vi "Create All Message Queues.vi"(8 "error in (no error)":errorcluster, 11 "Process Name":string) -> (0 "error out":errorcluster, 3 "Message Queues":T1)   [LabVIEW 2018, in "Feed Module.lvlib"]
uses:
  Feed Module.lvlib
  Controls/Feed Message Queues.ctl
  support/Message Queue/Message Cluster.ctl
  Config Module/Controls/OP Window Display.ctl
  Controls/Feed Module Display.ctl
  Measure Instrument/PID Input Enum.ctl
  Measure Instrument/PID 2 Output Enum.ctl
  support/Message Queue/Enqueue Message (Single).vi
  support/Message Queue/Message Queue.lvlib
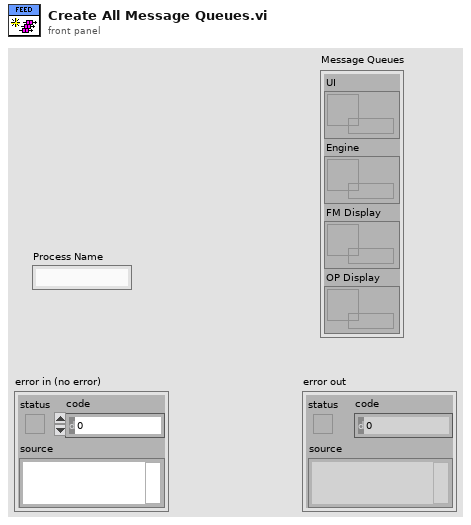
[diagram p1: front panel]
types:
  T1 = typedef "Feed Module.lvlib/Feed Message Queues.ctl" = cluster{"UI":refnum<queue>, "Engine":refnum<queue>, "FM Display":refnum<queue>, "OP Display":refnum<queue>}
  T2 = typedef "Feed Module.lvlib/Feed Module Display.ctl" = cluster{"Flow":dbl, "Density":dbl, "FL Temp":dbl, "Scale Value":dbl, "Pump On?":enum16{"Off", "On", "Not Initialized"}, "Cycle Period":dbl, "Input Device":T3, "Output":T4, "Pump's Pressure":dbl, "Pump's Flow ":dbl}
  T3 = typedef "PID Input Enum.ctl" = enum16{"Default", "Bronkhorst M13", "Bronkhorst M14", "Scale Rate of Change"}
  T4 = typedef "PID 2 Output Enum.ctl" = enum16{"Default", "Ismatec ISM 4308", "Ismatec ISM 831C", "Masterflex 7550-30", "VICI", "Tacmina QI", "KNF SIMDOS", "ASIA Type C", "FLOM UI-22-11", "SSI PR/LD", "SSI P40", "Masterflex 75211-70"}
  T5 = typedef "Feed Module.lvlib/OP Window Display.ctl" = cluster{"Flow":dbl, "Manual":dbl, "Pump Status":u16, "Smoothed Array":dbl[]}
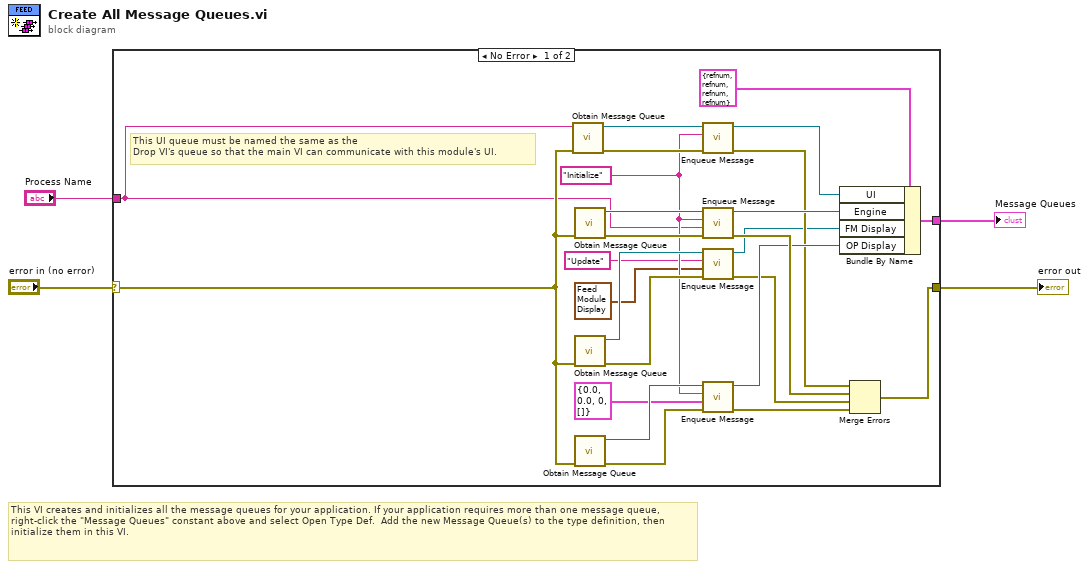
[diagram p0: block diagram]
diagram:
  # "This VI creates and initializes all the message queues for your application. If your application requires more than one message queue, right-click the \"Message Queues\" constant above and select Open Type Def.  Add the new Message Queue(s) to the type definition, then initialize them in this VI."
  n1 = case shown="No Error" "error in (no error)" {
    selector: "error in (no error)" -> [w15 w30]
    tunnel: [w26 w30] -> w4
    tunnel: [w29 _] -> w3
    tunnel: "Process Name" -> [w5 _]
    frame No Error {
      w12 = "Initialize" ("Message")
      # "This UI queue must be named the same as the \nDrop VI's queue so that the main VI can communicate with this module's UI."
      n2 = call "Obtain Message Queue.vi"("error in (no error)"=w15, "name (unnamed)"=w5) -> ("error out"=w28:errorcluster, "Message Queue"=w27:refnum<queue>)  [unwired: 8 in]
      n3 = call "Obtain Message Queue.vi"("error in (no error)"=w15) -> ("error out"=w24:errorcluster, "Message Queue"=w25:refnum<queue>)  [unwired: 9 in]
      n4 = call "Obtain Message Queue.vi"("error in (no error)"=w15) -> ("error out"=w21:errorcluster, "Message Queue"=w20:refnum<queue>)  [unwired: 9 in]
      n5 = call "Obtain Message Queue.vi"("error in (no error)"=w15) -> ("error out"=w19:errorcluster, "Message Queue"=w18:refnum<queue>)  [unwired: 9 in]
      n6 = call-poly "Enqueue Message.vi"("error in (no error)"=w28, "Message"=w12, "Message Queue"=w27) -> ("error out"=w10:errorcluster, "dup Message Queue"=w11:refnum<queue>)  [unwired: 7 in]
      n7 = call-poly "Enqueue Message.vi"("error in (no error)"=w24, "Message Data"=w5, "Message"=w12, "Message Queue"=w25) -> ("error out"=w22:errorcluster, "dup Message Queue"=w23:refnum<queue>)  [unwired: 6 in]
      n8 = call-poly "Enqueue Message.vi"("error in (no error)"=w21, "Message Data"=T2 {"Flow"=0.0, "Density"=0.0, "FL Temp"=0.0, "Scale Value"=0.0, "Pump On?"=enum."Not Initialized", "Cycle Period"=500.0, "Input Device"=enum."Default", "Output"=enum."Default", "Pump's Pressure"=0.0, "Pump's Flow "=0.0}, "Message"="Update", "Message Queue"=w20) -> ("error out"=w6:errorcluster, "dup Message Queue"=w7:refnum<queue>)  [unwired: 6 in]
      n9 = call-poly "Enqueue Message.vi"("error in (no error)"=w19, "Message Data"=T5 {"Flow"=0.0, "Manual"=0.0, "Pump Status"=0, "Smoothed Array"=[]}, "Message"=w12, "Message Queue"=w18) -> ("error out"=w13:errorcluster, "dup Message Queue"=w16:refnum<queue>)  [unwired: 6 in]
      n10 = Bundle By Name(cluster=T1 {"UI"=refnum, "Engine"=refnum, "FM Display"=refnum, "OP Display"=refnum} ("Message Queues"), "UI"=w11, "Engine"=w23, "FM Display"=w7, "OP Display"=w16) -> (w29:T1)
      n11 = Merge Errors(w10, w22, w6, w13) -> (w26:errorcluster)
    }
    frame Error {
    }
  }
  "Message Queues" <- w3
  "error out" <- w4
